vi "Slasher.vi"(1 "String In":string) -> (0 "String Out":string)   [LabVIEW 2014]
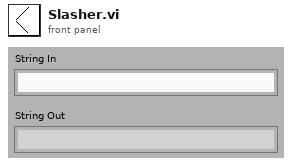
[diagram p1: front panel]
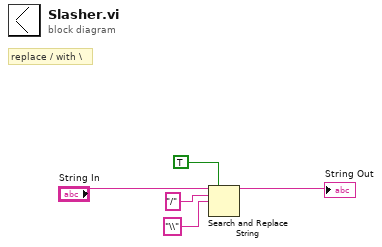
[diagram p0: block diagram]
diagram:
  # "replace / with \\"
  n1 = Search and Replace String(replace all?=TRUE ("replace all? (F)"), input string="String In", search string="/", replace string="\\" ("replace string (\"\")")) -> (result string=→"String Out":string)  [unwired: 4 in, 3 out]
